vi "ROI Settings from ini.vi"(7 "Section":string, 8 "error in (no error)":errorcluster, 10 "Operation":T1, 11 "Mask ROI In":T2={"left annulus"={"Center X"=929, "Center Y"=663, "Inner Radius"=200, "Outer Radius"=405, "Start Angle"=90.0, "End Angle"=180.0}, "right annulus"={"Center X"=929, "Center Y"=663, "Inner Radius"=200, "Outer Radius"=405, "Start Angle"=90.0, "End Angle"=180.0}, "Threshold Range"={"Lower value"=106.82432432432432, "Upper value"=255.0}, "[Avg BG]"=[0, 0, 0, 0, 0, 0, 0, 0, 0, 0, 0, 0, 0, 0, 0, 0, 0, 0, 0, 0, 0, 0, 0, 0, 0, 0, 0, 0, 0, 0, 0, 0], "Number of Sectors"=0, "Left ROI"={"Global Rectangle"=[], "Contours"=[]}, "Right ROI"={"Global Rectangle"=[], "Contours"=[]}, "Left Start Angle Duty Cycle"=0.0, "Left End Angle Duty Cycle"=0.0, "Right End Angle Duty Cycle"=0.0, "Right Start Angle Duty Cycle"=0.0, "[Sector ROIs]"=[], "Consecutive Sector Threshold"=0} {"[Sector ROIs]"."Contours"."Type" items=["No Selection", "Point", "Line", "Rectangle", "Oval", "Polygon", "Freehand Region", "Annulus", "Unused2", "Unused3", "Broken Line", "Freehand Line", "Rotated Rectangle"]; "Right ROI"."Contours"."Type" items=["No Selection", "Point", "Line", "Rectangle", "Oval", "Polygon", "Freehand Region", "Annulus", "Unused2", "Unused3", "Broken Line", "Freehand Line", "Rotated Rectangle"]; "Left ROI"."Contours"."Type" items=["No Selection", "Point", "Line", "Rectangle", "Oval", "Polygon", "Freehand Region", "Annulus", "Unused2", "Unused3", "Broken Line", "Freehand Line", "Rotated Rectangle"]; "Threshold Range"."Upper value" min=0.0 max=255.0 scale=0.0..255.0; "Threshold Range"."Lower value" min=0.0 max=255.0 scale=0.0..255.0; "right annulus"."End Angle" format="%.2f"; "right annulus"."Start Angle" format="%.2f"; "right annulus"."Center X" scale=0.0..1024.0; "left annulus"."End Angle" format="%.2f"; "left annulus"."Start Angle" format="%.2f"; "left annulus"."Center X" scale=0.0..1024.0}) -> (0 "error out":errorcluster, 3 "Mask ROI Out":T2={"left annulus"={"Center X"=929, "Center Y"=663, "Inner Radius"=200, "Outer Radius"=405, "Start Angle"=90.0, "End Angle"=180.0}, "right annulus"={"Center X"=929, "Center Y"=663, "Inner Radius"=200, "Outer Radius"=405, "Start Angle"=90.0, "End Angle"=180.0}, "Threshold Range"={"Lower value"=106.82432432432432, "Upper value"=255.0}, "[Avg BG]"=[], "Number of Sectors"=0, "Left ROI"={"Global Rectangle"=[], "Contours"=[]}, "Right ROI"={"Global Rectangle"=[], "Contours"=[]}, "Left Start Angle Duty Cycle"=0.0, "Left End Angle Duty Cycle"=0.0, "Right End Angle Duty Cycle"=0.0, "Right Start Angle Duty Cycle"=0.0, "[Sector ROIs]"=[], "Consecutive Sector Threshold"=0} {"[Sector ROIs]"."Contours"."Type" items=["No Selection", "Point", "Line", "Rectangle", "Oval", "Polygon", "Freehand Region", "Annulus", "Unused2", "Unused3", "Broken Line", "Freehand Line", "Rotated Rectangle"]; "Right ROI"."Contours"."Type" items=["No Selection", "Point", "Line", "Rectangle", "Oval", "Polygon", "Freehand Region", "Annulus", "Unused2", "Unused3", "Broken Line", "Freehand Line", "Rotated Rectangle"]; "Left ROI"."Contours"."Type" items=["No Selection", "Point", "Line", "Rectangle", "Oval", "Polygon", "Freehand Region", "Annulus", "Unused2", "Unused3", "Broken Line", "Freehand Line", "Rotated Rectangle"]; "Threshold Range"."Upper value" min=0.0 max=255.0 scale=0.0..255.0; "Threshold Range"."Lower value" min=0.0 max=255.0 scale=0.0..255.0; "right annulus"."End Angle" format="%.2f"; "right annulus"."Start Angle" format="%.2f"; "right annulus"."Center X" scale=0.0..1024.0; "left annulus"."End Angle" format="%.2f"; "left annulus"."Start Angle" format="%.2f"; "left annulus"."Center X" scale=0.0..1024.0}, 5 "All Tags Exists?":bool)   [LabVIEW 2013]
doc: "Loads the TCP port being used for listening for incoming connections."
uses:
  Image Processing/Mask ROI Cluster.ctl
  Common/File IO/INI/Read write mode.ctl
  ROI Setting Enum Keys.ctl
  Common/File IO/INI/INI Read write dbl.vi
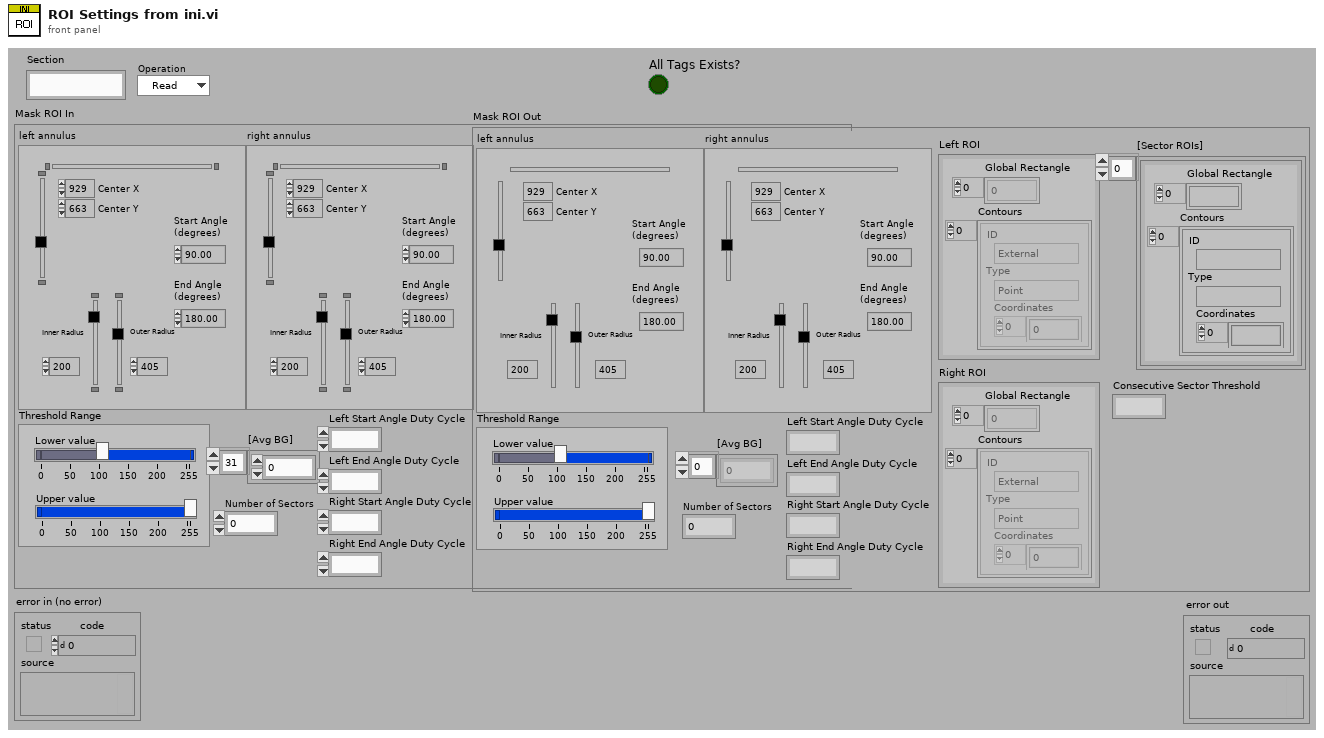
[diagram p1: front panel]
types:
  T1 = typedef "Read write mode.ctl" = enum16{"Read", "Write"}
  T2 = typedef "Mask ROI Cluster.ctl" = cluster{"left annulus":T3, "right annulus":T3, "Threshold Range":cluster{"Lower value":dbl, "Upper value":dbl}, "[Avg BG]":u8[], "Number of Sectors":u8, "Left ROI":T4, "Right ROI":T4, "Left Start Angle Duty Cycle":fxp<+,8,0>, "Left End Angle Duty Cycle":fxp<+,8,0>, "Right End Angle Duty Cycle":fxp<+,8,0>, "Right Start Angle Duty Cycle":fxp<+,8,0>, "[Sector ROIs]":T4[], "Consecutive Sector Threshold":u8}
  T3 = typedef "IMAQ Circle" = cluster{"Center X":i32, "Center Y":i32, "Inner Radius":i32, "Outer Radius":i32, "Start Angle":dbl, "End Angle":dbl}
  T4 = typedef "ROI Descriptor" = cluster{"Global Rectangle":i32[], "Contours":cluster{"ID":enum32{"External", "Internal"}, "Type":u32, "Coordinates":i32[]}[]}
  T5 = typedef "ROI Setting Enum Keys.ctl" = enum16{"Hinge Y", "Hinge X", "Start Angle", "End Angle", "Inner Radius", "Outer Radius", "Lower Threshold", "Sector BG", "Upper Threshold", "Number of Sectors", "Consecutive Sector Threshold"}
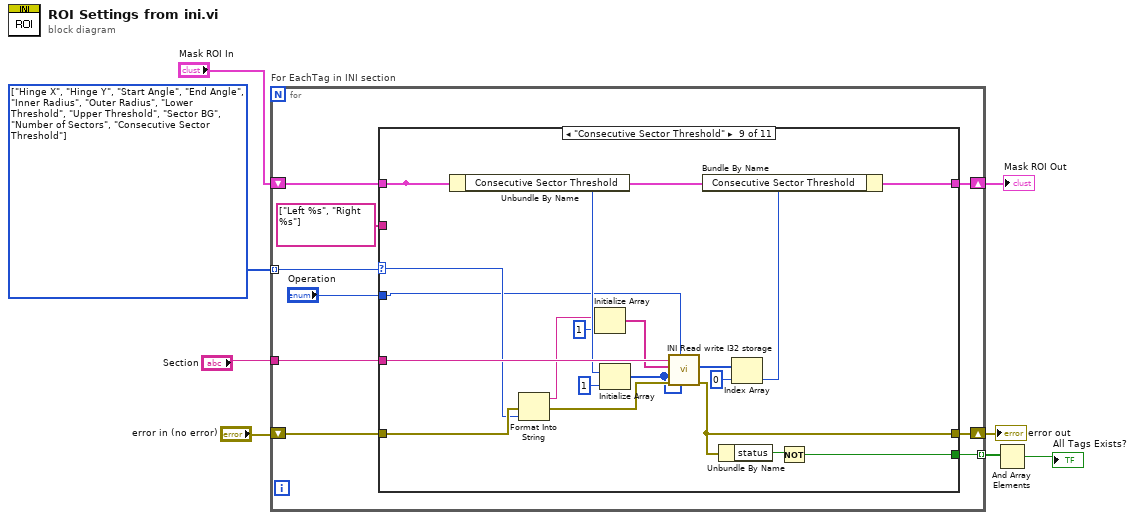
[diagram p0: block diagram]
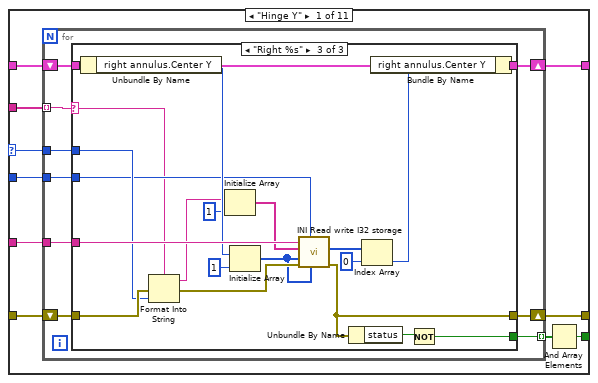
[diagram p2: hidden frame]
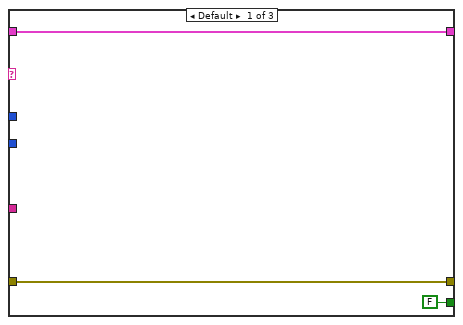
[diagram p3: hidden frame]
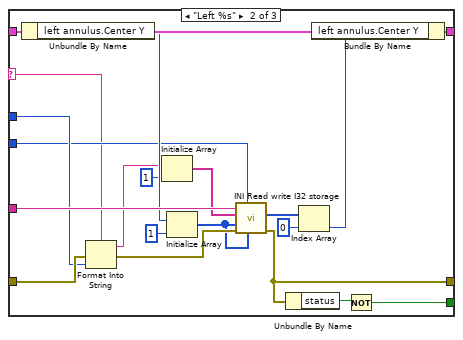
[diagram p4: hidden frame]
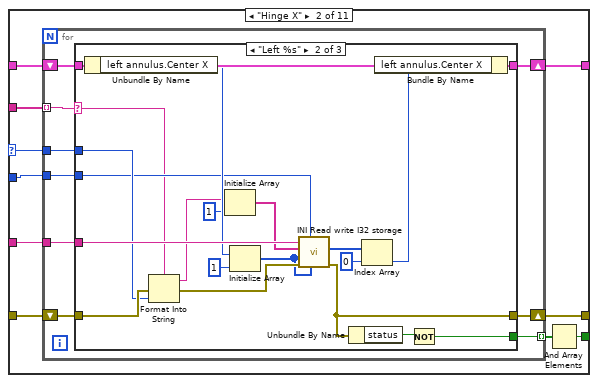
[diagram p5: hidden frame]
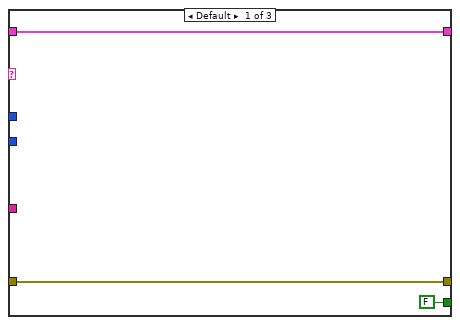
[diagram p6: hidden frame]
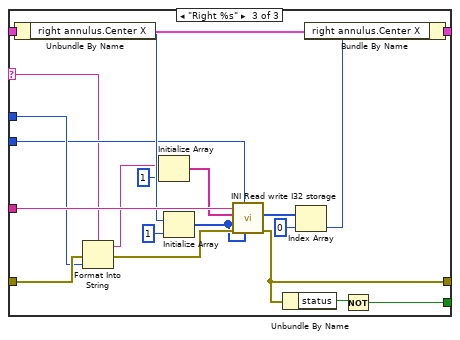
[diagram p7: hidden frame]
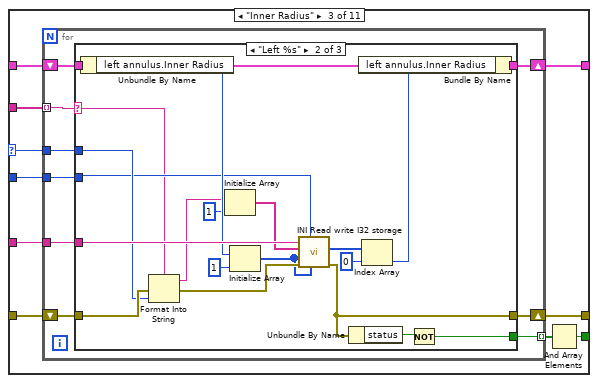
[diagram p8: hidden frame]
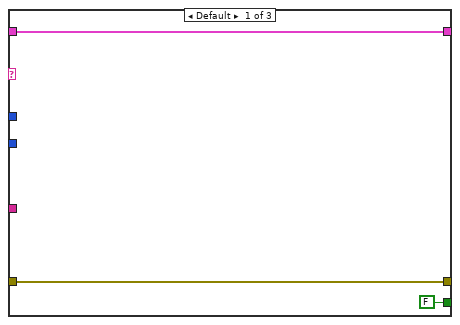
[diagram p9: hidden frame]
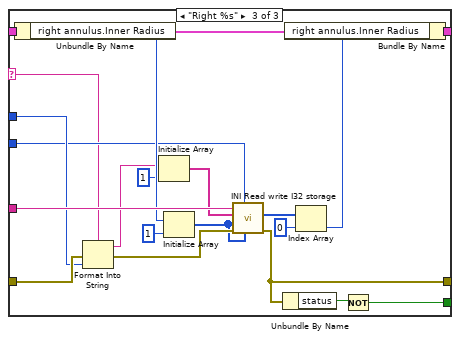
[diagram p10: hidden frame]
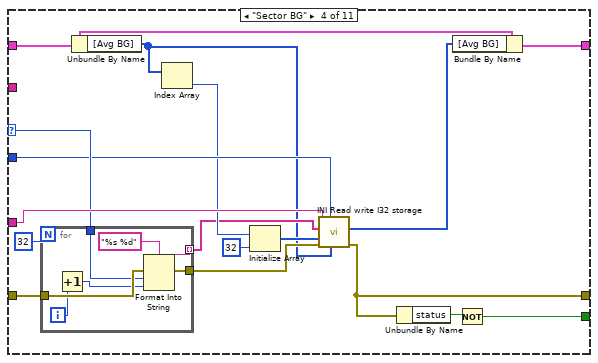
[diagram p11: hidden frame]
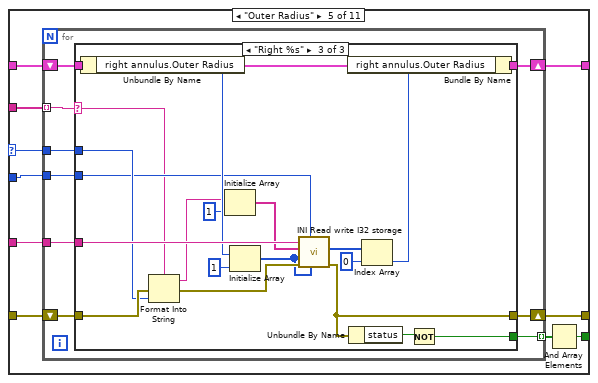
[diagram p12: hidden frame]
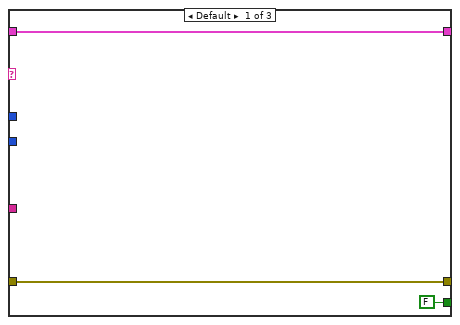
[diagram p13: hidden frame]
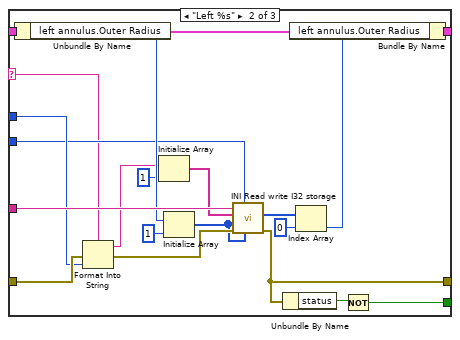
[diagram p14: hidden frame]
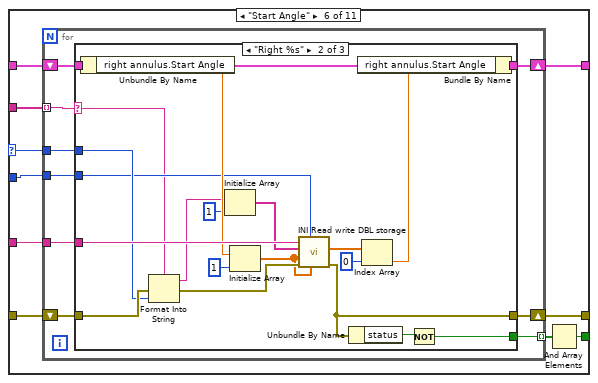
[diagram p15: hidden frame]
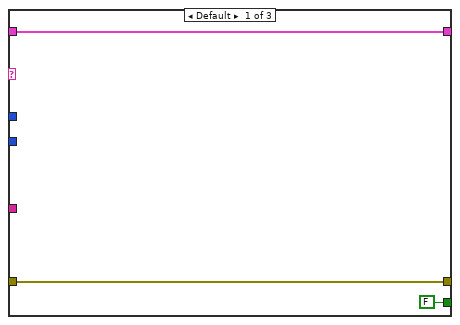
[diagram p16: hidden frame]
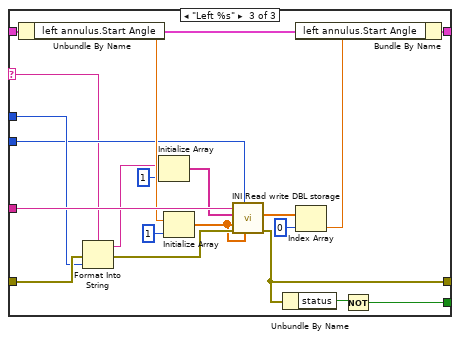
[diagram p17: hidden frame]
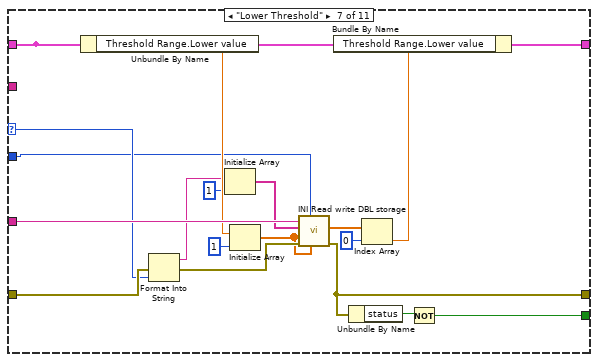
[diagram p18: hidden frame]
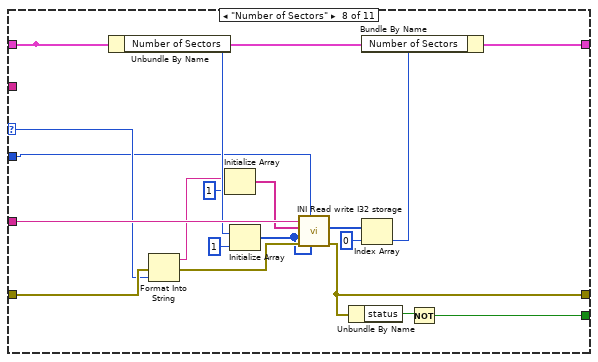
[diagram p19: hidden frame]
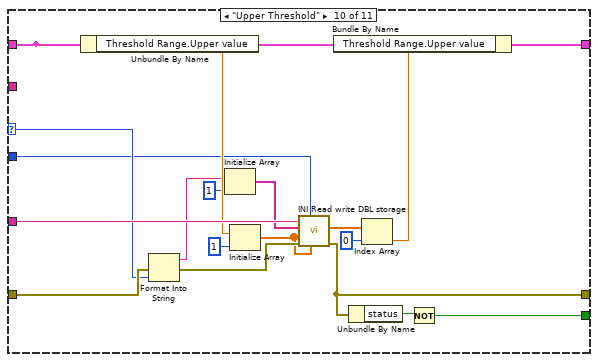
[diagram p20: hidden frame]
diagram:
  w8 = T5[] [enum."Hinge X", enum."Hinge Y", enum."Start Angle", enum."End Angle", enum."Inner Radius", enum."Outer Radius", enum."Lower Threshold", enum."Upper Threshold", enum."Sector BG", enum."Number of Sectors", enum."Consecutive Sector Threshold"] items=["Hinge Y", "Hinge X", "Start Angle", "End Angle", "Inner Radius", "Outer Radius", "Lower Threshold", "Sector BG", "Upper Threshold", "Number of Sectors", "Consecutive Sector Threshold"]
  n1 = for "For EachTag in INI section" {
    tunnel: "Section" -> [w17]
    tunnel: w8 -> [w11] mode=indexing
    shift-right: [w13] -> w6
    shift-left: "error in (no error)" -> [w15]
    shift-right: [w12] -> w1
    shift-left: "Mask ROI In" -> [w16]
    tunnel: [w14] -> w4 mode=indexing
    n2 = case shown="\"Consecutive Sector Threshold\"" w11 {
      selector: w11 -> [w22 w84 w146 w215 w232 w294 w365 w384 w403 w422 w432]
      tunnel: w17 -> [w26 w88 w150 w219 w236 w298 w369 w388 w407 w426 w436]
      tunnel: w16 -> [w24 w86 w148 w217 w234 w296 w367 w386 w405 w424 w434]
      tunnel: w15 -> [w23 w85 w147 w216 w233 w295 w366 w385 w404 w423 w433]
      tunnel: [w27 w89 w151 w220 w237 w299 w370 w389 w408 w427 w437] -> w13
      tunnel: [w19 w81 w143 w205 w229 w291 w354 w373 w392 w411 w429] -> w14
      tunnel: [w25 w87 w149 w218 w235 w297 w368 w387 w406 w425 w435] -> w12
      tunnel: string[] ["Left %s", "Right %s"] -> [w21 w83 w145 _ w231 w293 _ _ _ _ w431]
      tunnel: "Operation" -> [w18 w80 w142 w214 w228 w290 w352 w371 w390 w409 w428]
      frame "Hinge Y" {
        n3 = for {
          tunnel: w26 -> [w35]
          tunnel: w22 -> [w31]
          tunnel: [w30] -> w20 mode=indexing
          shift-right: [w34] -> w25
          shift-left: w24 -> [w33]
          tunnel: w21 -> [w29] mode=indexing
          shift-right: [w36] -> w27
          shift-left: w23 -> [w32]
          tunnel: w18 -> [w28]
          n4 = case shown="\"Right %s\"" w29 {
            selector: w29 -> [_ w40 w60]
            tunnel: [w37 w59 w79] -> w36
            tunnel: w35 -> [_ w58 w78]
            tunnel: [w39 w57 w77] -> w34
            tunnel: w33 -> [w39 w56 w76]
            tunnel: w32 -> [w37 w55 w75]
            tunnel: w31 -> [_ w54 w74]
            tunnel: [FALSE w43 w63] -> w30
            tunnel: w28 -> [_ w41 w61]
            frame Default {
            }
            frame "Left %s" {
              n5 = Unbundle By Name(w56) -> ("left annulus.Center Y"=w53:i32)
              n6 = Format Into String(format string=w40, error in=w55, w54) -> (resulting string=w51:string, error out=w44:errorcluster)  [unwired: 1 in]
              n7 = Initialize Array(w51, 1 ("dimension size")) -> (w49:string[])
              n8 = Initialize Array(w53, 1 ("dimension size")) -> (w42:i32[])
              n9 = call "INI Read write I32 storage.vi"("Values to write"=w42, "Read/Write mode"=w41, "error in"=w44, "Defaults"=w42, "keys"=w49, "section"=w58) -> ("error out"=w59:errorcluster, "Values"=w48:i32[])  [unwired: 4 in]
              n10 = Unbundle By Name(w59) -> ("status"=w45:bool)
              n11 = Index Array(array=w48, index=0) -> (element=w46:i32)
              n12 = Bundle By Name(cluster=w56, "left annulus.Center Y"=w46) -> (w57:T2)
              n13 = Not(x=w45) -> (.not. x?=w43:bool)
            }
            frame "Right %s" {
              n14 = Unbundle By Name(w76) -> ("right annulus.Center Y"=w73:i32)
              n15 = Format Into String(format string=w60, error in=w75, w74) -> (resulting string=w71:string, error out=w64:errorcluster)  [unwired: 1 in]
              n16 = Initialize Array(w71, 1 ("dimension size")) -> (w69:string[])
              n17 = Initialize Array(w73, 1 ("dimension size")) -> (w62:i32[])
              n18 = call "INI Read write I32 storage.vi"("Values to write"=w62, "Read/Write mode"=w61, "error in"=w64, "Defaults"=w62, "keys"=w69, "section"=w78) -> ("error out"=w79:errorcluster, "Values"=w68:i32[])  [unwired: 4 in]
              n19 = Unbundle By Name(w79) -> ("status"=w65:bool)
              n20 = Index Array(array=w68, index=0) -> (element=w66:i32)
              n21 = Bundle By Name(cluster=w76, "right annulus.Center Y"=w66) -> (w77:T2)
              n22 = Not(x=w65) -> (.not. x?=w63:bool)
            }
          }
        }
        n23 = And Array Elements(Boolean array=w20) -> (logical AND=w19:bool)
      }
      frame "Hinge X" {
        n24 = for {
          tunnel: w88 -> [w97]
          tunnel: w84 -> [w93]
          tunnel: [w92] -> w82 mode=indexing
          shift-right: [w96] -> w87
          shift-left: w86 -> [w95]
          tunnel: w83 -> [w91] mode=indexing
          shift-right: [w98] -> w89
          shift-left: w85 -> [w94]
          tunnel: w80 -> [w90]
          n25 = case shown="\"Left %s\"" w91 {
            selector: w91 -> [_ w102 w122]
            tunnel: [w99 w121 w141] -> w98
            tunnel: w97 -> [_ w120 w140]
            tunnel: [w101 w119 w139] -> w96
            tunnel: w95 -> [w101 w118 w138]
            tunnel: w94 -> [w99 w117 w137]
            tunnel: w93 -> [_ w116 w136]
            tunnel: [FALSE w105 w125] -> w92
            tunnel: w90 -> [_ w103 w123]
            frame Default {
            }
            frame "Left %s" {
              n26 = Unbundle By Name(w118) -> ("left annulus.Center X"=w115:i32)
              n27 = Format Into String(format string=w102, error in=w117, w116) -> (resulting string=w113:string, error out=w106:errorcluster)  [unwired: 1 in]
              n28 = Initialize Array(w113, 1 ("dimension size")) -> (w111:string[])
              n29 = Initialize Array(w115, 1 ("dimension size")) -> (w104:i32[])
              n30 = call "INI Read write I32 storage.vi"("Values to write"=w104, "Read/Write mode"=w103, "error in"=w106, "Defaults"=w104, "keys"=w111, "section"=w120) -> ("error out"=w121:errorcluster, "Values"=w110:i32[])  [unwired: 4 in]
              n31 = Unbundle By Name(w121) -> ("status"=w107:bool)
              n32 = Index Array(array=w110, index=0) -> (element=w108:i32)
              n33 = Bundle By Name(cluster=w118, "left annulus.Center X"=w108) -> (w119:T2)
              n34 = Not(x=w107) -> (.not. x?=w105:bool)
            }
            frame "Right %s" {
              n35 = Unbundle By Name(w138) -> ("right annulus.Center X"=w135:i32)
              n36 = Format Into String(format string=w122, error in=w137, w136) -> (resulting string=w133:string, error out=w126:errorcluster)  [unwired: 1 in]
              n37 = Initialize Array(w133, 1 ("dimension size")) -> (w131:string[])
              n38 = Initialize Array(w135, 1 ("dimension size")) -> (w124:i32[])
              n39 = call "INI Read write I32 storage.vi"("Values to write"=w124, "Read/Write mode"=w123, "error in"=w126, "Defaults"=w124, "keys"=w131, "section"=w140) -> ("error out"=w141:errorcluster, "Values"=w130:i32[])  [unwired: 4 in]
              n40 = Unbundle By Name(w141) -> ("status"=w127:bool)
              n41 = Index Array(array=w130, index=0) -> (element=w128:i32)
              n42 = Bundle By Name(cluster=w138, "right annulus.Center X"=w128) -> (w139:T2)
              n43 = Not(x=w127) -> (.not. x?=w125:bool)
            }
          }
        }
        n44 = And Array Elements(Boolean array=w82) -> (logical AND=w81:bool)
      }
      frame "Inner Radius" {
        n45 = for {
          tunnel: w150 -> [w159]
          tunnel: w146 -> [w155]
          tunnel: [w154] -> w144 mode=indexing
          shift-right: [w158] -> w149
          shift-left: w148 -> [w157]
          tunnel: w145 -> [w153] mode=indexing
          shift-right: [w160] -> w151
          shift-left: w147 -> [w156]
          tunnel: w142 -> [w152]
          n46 = case shown="\"Left %s\"" w153 {
            selector: w153 -> [_ w164 w184]
            tunnel: [w161 w183 w203] -> w160
            tunnel: w159 -> [_ w182 w202]
            tunnel: [w163 w181 w201] -> w158
            tunnel: w157 -> [w163 w180 w200]
            tunnel: w156 -> [w161 w179 w199]
            tunnel: w155 -> [_ w178 w198]
            tunnel: [FALSE w167 w187] -> w154
            tunnel: w152 -> [_ w165 w185]
            frame Default {
            }
            frame "Left %s" {
              n47 = Unbundle By Name(w180) -> ("left annulus.Inner Radius"=w177:i32)
              n48 = Format Into String(format string=w164, error in=w179, w178) -> (resulting string=w175:string, error out=w168:errorcluster)  [unwired: 1 in]
              n49 = Initialize Array(w175, 1 ("dimension size")) -> (w173:string[])
              n50 = Initialize Array(w177, 1 ("dimension size")) -> (w166:i32[])
              n51 = call "INI Read write I32 storage.vi"("Values to write"=w166, "Read/Write mode"=w165, "error in"=w168, "Defaults"=w166, "keys"=w173, "section"=w182) -> ("error out"=w183:errorcluster, "Values"=w172:i32[])  [unwired: 4 in]
              n52 = Unbundle By Name(w183) -> ("status"=w169:bool)
              n53 = Index Array(array=w172, index=0) -> (element=w170:i32)
              n54 = Bundle By Name(cluster=w180, "left annulus.Inner Radius"=w170) -> (w181:T2)
              n55 = Not(x=w169) -> (.not. x?=w167:bool)
            }
            frame "Right %s" {
              n56 = Unbundle By Name(w200) -> ("right annulus.Inner Radius"=w197:i32)
              n57 = Format Into String(format string=w184, error in=w199, w198) -> (resulting string=w195:string, error out=w188:errorcluster)  [unwired: 1 in]
              n58 = Initialize Array(w195, 1 ("dimension size")) -> (w193:string[])
              n59 = Initialize Array(w197, 1 ("dimension size")) -> (w186:i32[])
              n60 = call "INI Read write I32 storage.vi"("Values to write"=w186, "Read/Write mode"=w185, "error in"=w188, "Defaults"=w186, "keys"=w193, "section"=w202) -> ("error out"=w203:errorcluster, "Values"=w192:i32[])  [unwired: 4 in]
              n61 = Unbundle By Name(w203) -> ("status"=w189:bool)
              n62 = Index Array(array=w192, index=0) -> (element=w190:i32)
              n63 = Bundle By Name(cluster=w200, "right annulus.Inner Radius"=w190) -> (w201:T2)
              n64 = Not(x=w189) -> (.not. x?=w187:bool)
            }
          }
        }
        n65 = And Array Elements(Boolean array=w144) -> (logical AND=w143:bool)
      }
      frame "Sector BG" {
        n66 = for {
          N: 32 -> [_]
          tunnel: w216 -> [w227]
          tunnel: w215 -> [w226]
          tunnel: [w225] -> w211
          tunnel: [w222] -> w207 mode=indexing
          i -> [w221]
          n67 = Increment(x=w221) -> (x+1=w223:i32)
          n68 = Format Into String(format string="%s %d", error in=w227, w226, w223) -> (resulting string=w222:string, error out=w225:errorcluster)  [unwired: 1 in]
        }
        n69 = Unbundle By Name(w217) -> ("[Avg BG]"=w204:u8[])
        n70 = Index Array(array=w204) -> (element=w209:u8)  [unwired: 1 in]
        n71 = Initialize Array(w209, 32 ("dimension size")) -> (w210:u8[])
        n72 = call "INI Read write I32 storage.vi"("Values to write"=w204, "Read/Write mode"=w214, "error in"=w211, "Defaults"=w210, "keys"=w207, "section"=w219) -> ("error out"=w220:errorcluster, "Values"=w206:i32[])  [unwired: 4 in]
        n73 = Unbundle By Name(w220) -> ("status"=w212:bool)
        n74 = Bundle By Name(cluster=w217, "[Avg BG]"=w206) -> (w218:T2)
        n75 = Not(x=w212) -> (.not. x?=w205:bool)
      }
      frame "Outer Radius" {
        n76 = for {
          tunnel: w236 -> [w245]
          tunnel: w232 -> [w241]
          tunnel: [w240] -> w230 mode=indexing
          shift-right: [w244] -> w235
          shift-left: w234 -> [w243]
          tunnel: w231 -> [w239] mode=indexing
          shift-right: [w246] -> w237
          shift-left: w233 -> [w242]
          tunnel: w228 -> [w238]
          n77 = case shown="\"Right %s\"" w239 {
            selector: w239 -> [_ w250 w270]
            tunnel: [w247 w269 w289] -> w246
            tunnel: w245 -> [_ w268 w288]
            tunnel: [w249 w267 w287] -> w244
            tunnel: w243 -> [w249 w266 w286]
            tunnel: w242 -> [w247 w265 w285]
            tunnel: w241 -> [_ w264 w284]
            tunnel: [FALSE w253 w273] -> w240
            tunnel: w238 -> [_ w251 w271]
            frame Default {
            }
            frame "Left %s" {
              n78 = Unbundle By Name(w266) -> ("left annulus.Outer Radius"=w263:i32)
              n79 = Format Into String(format string=w250, error in=w265, w264) -> (resulting string=w261:string, error out=w254:errorcluster)  [unwired: 1 in]
              n80 = Initialize Array(w261, 1 ("dimension size")) -> (w259:string[])
              n81 = Initialize Array(w263, 1 ("dimension size")) -> (w252:i32[])
              n82 = call "INI Read write I32 storage.vi"("Values to write"=w252, "Read/Write mode"=w251, "error in"=w254, "Defaults"=w252, "keys"=w259, "section"=w268) -> ("error out"=w269:errorcluster, "Values"=w258:i32[])  [unwired: 4 in]
              n83 = Unbundle By Name(w269) -> ("status"=w255:bool)
              n84 = Index Array(array=w258, index=0) -> (element=w256:i32)
              n85 = Bundle By Name(cluster=w266, "left annulus.Outer Radius"=w256) -> (w267:T2)
              n86 = Not(x=w255) -> (.not. x?=w253:bool)
            }
            frame "Right %s" {
              n87 = Unbundle By Name(w286) -> ("right annulus.Outer Radius"=w283:i32)
              n88 = Format Into String(format string=w270, error in=w285, w284) -> (resulting string=w281:string, error out=w274:errorcluster)  [unwired: 1 in]
              n89 = Initialize Array(w281, 1 ("dimension size")) -> (w279:string[])
              n90 = Initialize Array(w283, 1 ("dimension size")) -> (w272:i32[])
              n91 = call "INI Read write I32 storage.vi"("Values to write"=w272, "Read/Write mode"=w271, "error in"=w274, "Defaults"=w272, "keys"=w279, "section"=w288) -> ("error out"=w289:errorcluster, "Values"=w278:i32[])  [unwired: 4 in]
              n92 = Unbundle By Name(w289) -> ("status"=w275:bool)
              n93 = Index Array(array=w278, index=0) -> (element=w276:i32)
              n94 = Bundle By Name(cluster=w286, "right annulus.Outer Radius"=w276) -> (w287:T2)
              n95 = Not(x=w275) -> (.not. x?=w273:bool)
            }
          }
        }
        n96 = And Array Elements(Boolean array=w230) -> (logical AND=w229:bool)
      }
      frame "Start Angle" {
        n97 = for {
          tunnel: w298 -> [w307]
          tunnel: w294 -> [w303]
          tunnel: [w302] -> w292 mode=indexing
          shift-right: [w306] -> w297
          shift-left: w296 -> [w305]
          tunnel: w293 -> [w301] mode=indexing
          shift-right: [w308] -> w299
          shift-left: w295 -> [w304]
          tunnel: w290 -> [w300]
          n98 = case shown="\"Right %s\"" w301 {
            selector: w301 -> [_ w312 w332]
            tunnel: [w309 w331 w351] -> w308
            tunnel: w307 -> [_ w330 w350]
            tunnel: [w311 w329 w349] -> w306
            tunnel: w305 -> [w311 w328 w348]
            tunnel: w304 -> [w309 w327 w347]
            tunnel: w303 -> [_ w326 w346]
            tunnel: [FALSE w315 w335] -> w302
            tunnel: w300 -> [_ w313 w333]
            frame Default {
            }
            frame "Right %s" {
              n99 = Unbundle By Name(w328) -> ("right annulus.Start Angle"=w325:dbl)
              n100 = Format Into String(format string=w312, error in=w327, w326) -> (resulting string=w323:string, error out=w316:errorcluster)  [unwired: 1 in]
              n101 = Initialize Array(w323, 1 ("dimension size")) -> (w321:string[])
              n102 = Initialize Array(w325, 1 ("dimension size")) -> (w314:dbl[])
              n103 = call "INI Read write DBL storage.vi"("Values to write"=w314, "Read/Write mode"=w313, "error in"=w316, "Default"=w314, "keys"=w321, "section"=w330) -> ("error out"=w331:errorcluster, "Values"=w320:dbl[])  [unwired: 4 in]
              n104 = Unbundle By Name(w331) -> ("status"=w317:bool)
              n105 = Index Array(array=w320, index=0) -> (element=w318:dbl)
              n106 = Bundle By Name(cluster=w328, "right annulus.Start Angle"=w318) -> (w329:T2)
              n107 = Not(x=w317) -> (.not. x?=w315:bool)
            }
            frame "Left %s" {
              n108 = Unbundle By Name(w348) -> ("left annulus.Start Angle"=w345:dbl)
              n109 = Format Into String(format string=w332, error in=w347, w346) -> (resulting string=w343:string, error out=w336:errorcluster)  [unwired: 1 in]
              n110 = Initialize Array(w343, 1 ("dimension size")) -> (w341:string[])
              n111 = Initialize Array(w345, 1 ("dimension size")) -> (w334:dbl[])
              n112 = call "INI Read write DBL storage.vi"("Values to write"=w334, "Read/Write mode"=w333, "error in"=w336, "Default"=w334, "keys"=w341, "section"=w350) -> ("error out"=w351:errorcluster, "Values"=w340:dbl[])  [unwired: 4 in]
              n113 = Unbundle By Name(w351) -> ("status"=w337:bool)
              n114 = Index Array(array=w340, index=0) -> (element=w338:dbl)
              n115 = Bundle By Name(cluster=w348, "left annulus.Start Angle"=w338) -> (w349:T2)
              n116 = Not(x=w337) -> (.not. x?=w335:bool)
            }
          }
        }
        n117 = And Array Elements(Boolean array=w292) -> (logical AND=w291:bool)
      }
      frame "Lower Threshold" {
        n118 = Unbundle By Name(w367) -> ("Threshold Range.Lower value"=w364:dbl)
        n119 = Format Into String(error in=w366, w365) -> (resulting string=w362:string, error out=w355:errorcluster)  [unwired: 2 in]
        n120 = Initialize Array(w362, 1 ("dimension size")) -> (w360:string[])
        n121 = Initialize Array(w364, 1 ("dimension size")) -> (w353:dbl[])
        n122 = call "INI Read write DBL storage.vi"("Values to write"=w353, "Read/Write mode"=w352, "error in"=w355, "Default"=w353, "keys"=w360, "section"=w369) -> ("error out"=w370:errorcluster, "Values"=w359:dbl[])  [unwired: 4 in]
        n123 = Unbundle By Name(w370) -> ("status"=w356:bool)
        n124 = Index Array(array=w359, index=0) -> (element=w357:dbl)
        n125 = Bundle By Name(cluster=w367, "Threshold Range.Lower value"=w357) -> (w368:T2)
        n126 = Not(x=w356) -> (.not. x?=w354:bool)
      }
      frame "Number of Sectors" {
        n127 = Unbundle By Name(w386) -> ("Number of Sectors"=w383:u8)
        n128 = Format Into String(error in=w385, w384) -> (resulting string=w381:string, error out=w374:errorcluster)  [unwired: 2 in]
        n129 = Initialize Array(w381, 1 ("dimension size")) -> (w379:string[])
        n130 = Initialize Array(w383, 1 ("dimension size")) -> (w372:u8[])
        n131 = call "INI Read write I32 storage.vi"("Values to write"=w372, "Read/Write mode"=w371, "error in"=w374, "Defaults"=w372, "keys"=w379, "section"=w388) -> ("error out"=w389:errorcluster, "Values"=w378:i32[])  [unwired: 4 in]
        n132 = Unbundle By Name(w389) -> ("status"=w375:bool)
        n133 = Index Array(array=w378, index=0) -> (element=w376:i32)
        n134 = Bundle By Name(cluster=w386, "Number of Sectors"=w376) -> (w387:T2)
        n135 = Not(x=w375) -> (.not. x?=w373:bool)
      }
      frame "Consecutive Sector Threshold" {
        n136 = Unbundle By Name(w405) -> ("Consecutive Sector Threshold"=w402:u8)
        n137 = Format Into String(error in=w404, w403) -> (resulting string=w400:string, error out=w393:errorcluster)  [unwired: 2 in]
        n138 = Initialize Array(w400, 1 ("dimension size")) -> (w398:string[])
        n139 = Initialize Array(w402, 1 ("dimension size")) -> (w391:u8[])
        n140 = call "INI Read write I32 storage.vi"("Values to write"=w391, "Read/Write mode"=w390, "error in"=w393, "Defaults"=w391, "keys"=w398, "section"=w407) -> ("error out"=w408:errorcluster, "Values"=w397:i32[])  [unwired: 4 in]
        n141 = Unbundle By Name(w408) -> ("status"=w394:bool)
        n142 = Index Array(array=w397, index=0) -> (element=w395:i32)
        n143 = Bundle By Name(cluster=w405, "Consecutive Sector Threshold"=w395) -> (w406:T2)
        n144 = Not(x=w394) -> (.not. x?=w392:bool)
      }
      frame "Upper Threshold" {
        n145 = Unbundle By Name(w424) -> ("Threshold Range.Upper value"=w421:dbl)
        n146 = Format Into String(error in=w423, w422) -> (resulting string=w419:string, error out=w412:errorcluster)  [unwired: 2 in]
        n147 = Initialize Array(w419, 1 ("dimension size")) -> (w417:string[])
        n148 = Initialize Array(w421, 1 ("dimension size")) -> (w410:dbl[])
        n149 = call "INI Read write DBL storage.vi"("Values to write"=w410, "Read/Write mode"=w409, "error in"=w412, "Default"=w410, "keys"=w417, "section"=w426) -> ("error out"=w427:errorcluster, "Values"=w416:dbl[])  [unwired: 4 in]
        n150 = Unbundle By Name(w427) -> ("status"=w413:bool)
        n151 = Index Array(array=w416, index=0) -> (element=w414:dbl)
        n152 = Bundle By Name(cluster=w424, "Threshold Range.Upper value"=w414) -> (w425:T2)
        n153 = Not(x=w413) -> (.not. x?=w411:bool)
      }
      frame "End Angle" {
        n154 = for {
          tunnel: w436 -> [w445]
          tunnel: w432 -> [w441]
          tunnel: [w440] -> w430 mode=indexing
          shift-right: [w444] -> w435
          shift-left: w434 -> [w443]
          tunnel: w431 -> [w439] mode=indexing
          shift-right: [w446] -> w437
          shift-left: w433 -> [w442]
          tunnel: w428 -> [w438]
          n155 = case shown="\"Right %s\"" w439 {
            selector: w439 -> [_ w450 w470]
            tunnel: [w447 w469 w489] -> w446
            tunnel: w445 -> [_ w468 w488]
            tunnel: [w449 w467 w487] -> w444
            tunnel: w443 -> [w449 w466 w486]
            tunnel: w442 -> [w447 w465 w485]
            tunnel: w441 -> [_ w464 w484]
            tunnel: [FALSE w453 w473] -> w440
            tunnel: w438 -> [_ w451 w471]
            frame Default {
            }
            frame "Right %s" {
              n156 = Unbundle By Name(w466) -> ("right annulus.End Angle"=w463:dbl)
              n157 = Format Into String(format string=w450, error in=w465, w464) -> (resulting string=w461:string, error out=w454:errorcluster)  [unwired: 1 in]
              n158 = Initialize Array(w461, 1 ("dimension size")) -> (w459:string[])
              n159 = Initialize Array(w463, 1 ("dimension size")) -> (w452:dbl[])
              n160 = call "INI Read write DBL storage.vi"("Values to write"=w452, "Read/Write mode"=w451, "error in"=w454, "Default"=w452, "keys"=w459, "section"=w468) -> ("error out"=w469:errorcluster, "Values"=w458:dbl[])  [unwired: 4 in]
              n161 = Unbundle By Name(w469) -> ("status"=w455:bool)
              n162 = Index Array(array=w458, index=0) -> (element=w456:dbl)
              n163 = Bundle By Name(cluster=w466, "right annulus.End Angle"=w456) -> (w467:T2)
              n164 = Not(x=w455) -> (.not. x?=w453:bool)
            }
            frame "Left %s" {
              n165 = Unbundle By Name(w486) -> ("left annulus.End Angle"=w483:dbl)
              n166 = Format Into String(format string=w470, error in=w485, w484) -> (resulting string=w481:string, error out=w474:errorcluster)  [unwired: 1 in]
              n167 = Initialize Array(w481, 1 ("dimension size")) -> (w479:string[])
              n168 = Initialize Array(w483, 1 ("dimension size")) -> (w472:dbl[])
              n169 = call "INI Read write DBL storage.vi"("Values to write"=w472, "Read/Write mode"=w471, "error in"=w474, "Default"=w472, "keys"=w479, "section"=w488) -> ("error out"=w489:errorcluster, "Values"=w478:dbl[])  [unwired: 4 in]
              n170 = Unbundle By Name(w489) -> ("status"=w475:bool)
              n171 = Index Array(array=w478, index=0) -> (element=w476:dbl)
              n172 = Bundle By Name(cluster=w486, "left annulus.End Angle"=w476) -> (w487:T2)
              n173 = Not(x=w475) -> (.not. x?=w473:bool)
            }
          }
        }
        n174 = And Array Elements(Boolean array=w430) -> (logical AND=w429:bool)
      }
    }
  }
  "error out" <- w6
  "Mask ROI Out" <- w1
  n175 = And Array Elements(Boolean array=w4) -> (logical AND=→"All Tags Exists?":bool)
